vi "Get Device.vi"() -> (1 "Device":T1)   [LabVIEW 2021]
uses:
  Type Definitions/Device.ctl
  Type Definitions/Device Parameters.ctl
  Type Definitions/Data Frame.ctl
  Type Definitions/Data Frame Header.ctl
  Type Definitions/Payload Class.ctl
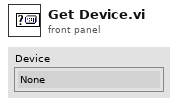
[diagram p1: front panel]
types:
  T1 = typedef "Device.ctl" = enum32{"None", "Exec", "Aux1", "Aux2", "Aux3"}
  T2 = typedef "Data Frame.ctl" = cluster{"Frame Header":T3, "Payload":string, "CRC":u32}
  T3 = typedef "Data Frame Header.ctl" = cluster{"Sync":u32, "Time":dbl, "Nanosecond Counter":i64, "Payload Class":T4, "Payload ID":u16, "Counter":i32, "Options":u32, "Source":T1, "Destination":T1}
  T4 = typedef "Payload Class.ctl" = enum16{"System State", "Parameters", "Metadata", "Software Monitor", "Data", "Commands"}
  T5 = typedef "Device Parameters.ctl" = cluster{"Device":T1}
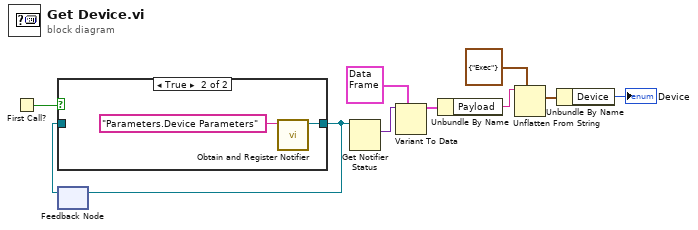
[diagram p0: block diagram]
diagram:
  n1 = First Call?() -> (First Call?: T/F=w10:bool)
  n2 = feedback #1() -> (w9:refnum<notifier>)  [unwired: 1 in]
  n3 = case shown="True" w10 {
    tunnel: w9 -> [w11 _]
    tunnel: [w11 w12] -> w1
    frame False {
    }
    frame True {
      n4 = call "Obtain and Register Notifier.vi"("name (unnamed)"="Parameters.Device Parameters") -> ("notifier out"=w12:refnum<notifier>)  [unwired: 8 in, 2 out]
    }
  }
  n5 = feedback-in #1(w1) -> ()
  n6 = Get Notifier Status(notifier=w1) -> (current notification=w8:variant)  [unwired: 1 in, 4 out]
  n7 = Variant To Data(type=T2 {"Frame Header"={"Sync"=0, "Time"=0.0, "Nanosecond Counter"=0, "Payload Class"=enum."System State", "Payload ID"=0, "Counter"=0, "Options"=0, "Source"=enum."None", "Destination"=enum."None"}, "Payload"="", "CRC"=0} ("Frame"), Variant=w8) -> (data=w7:T2)  [unwired: 1 in, 1 out]
  n8 = Unbundle By Name(w7) -> ("Payload"=w6:string)
  n9 = Unflatten From String(type=T5 {"Device"=enum."Exec"} ("Device Parameters"), binary string=w6) -> (value=w5:T5)  [unwired: 3 in, 2 out]
  n10 = Unbundle By Name(w5) -> ("Device"=→"Device":T1)
